vi "HGF_DSCmonitor_deregister.vi"(0 "HGF_DSCMonitor in":refnum<class "HGF_DSCMonitor.lvclass">, 1 "SV":refnum<k21>, 3 "HGF_NetworkVisitor":refnum<class "HGF_NetworkVisitor.lvclass">, 4 "HGF_TriggeredEvent":refnum<class "HGF_TriggeredEvent.lvclass">, 5 "error in (no error)":errorcluster, 9 "Rem SV/Visitor from List":bool) -> (14 "HGF_DSCMonitor out":refnum<class "HGF_DSCMonitor.lvclass">, 19 "error out":errorcluster)   [LabVIEW 2012, in "HGF_DSC.lvlib" / "HGF_DSCMonitor.lvclass"]
uses:
  HGF_DSCMonitor.lvclass
  HGF_BaseClasses/HGF_NetworkVisitor/HGF_NetworkVisitor.lvclass
  HGF_BaseClasses/HGF_TriggeredEvent/HGF_TriggeredEvent.lvclass
  HGF_DSCMonitor.lvclass/HGF_DSCMonitor.ctl
  <vilib>/lvdsc/NI_DSC.lvlib
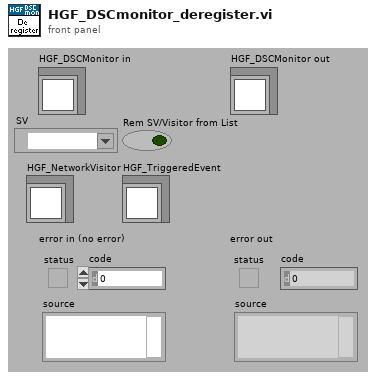
[diagram p1: front panel]
types:
  T1 = cluster{"Shared Variable":refnum<k21>, "registered Visitors":cluster{"HGF_NetworkVisitor":refnum<class "HGF_NetworkVisitor.lvclass">, "HGF_TriggeredEvent":refnum<class "HGF_TriggeredEvent.lvclass">}[]}[]
  T2 = cluster{"HGF_NetworkVisitor":refnum<class "HGF_NetworkVisitor.lvclass">, "HGF_TriggeredEvent":refnum<class "HGF_TriggeredEvent.lvclass">}
  T3 = cluster{"Shared Variable":refnum<k21>, "registered Visitors":cluster{"HGF_NetworkVisitor":refnum<class "HGF_NetworkVisitor.lvclass">, "HGF_TriggeredEvent":refnum<class "HGF_TriggeredEvent.lvclass">}[]}
  T4 = cluster{"HGF_NetworkVisitor":refnum<class "HGF_NetworkVisitor.lvclass">, "HGF_TriggeredEvent":refnum<class "HGF_TriggeredEvent.lvclass">}[]
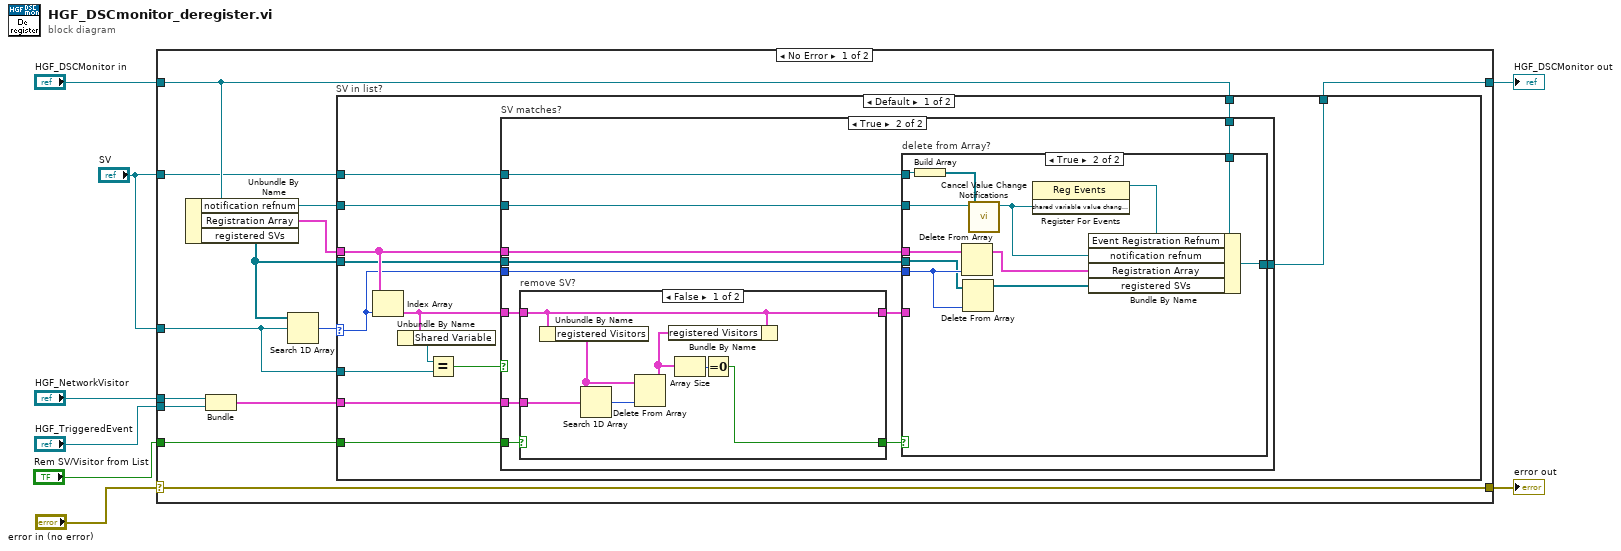
[diagram p0: block diagram]
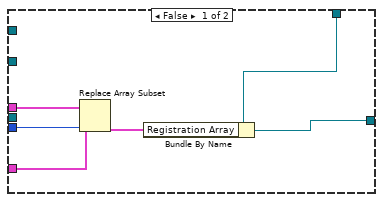
[diagram p3: hidden frame]
diagram:
  n1 = case shown="No Error" "error in (no error)" {
    selector: "error in (no error)" -> [w21 w76]
    tunnel: [w21 w76] -> w7
    tunnel: [w11 w75] -> w5
    tunnel: "HGF_DSCMonitor in" -> [w12 w75]
    tunnel: "SV" -> [w16 _]
    tunnel: "HGF_TriggeredEvent" -> [w18 _]
    tunnel: "HGF_NetworkVisitor" -> [w17 _]
    tunnel: "Rem SV/Visitor from List" -> [w14 _]
    tunnel: "SV" -> [w9 _]
    frame No Error {
      n2 = Unbundle By Name(w12) -> ("notification refnum"=w10:refnum<user-event>, "Registration Array"=w19:T1, "registered SVs"=w13:refnum<k21>[])
      n3 = Bundle("HGF_NetworkVisitor"=w17, "HGF_TriggeredEvent"=w18) -> (w15:T2)  [unwired: 1 out]
      n4 = Search 1D Array(1D array=w13, element=w16) -> (index of element=w20:i32)  [unwired: 1 out]
      n5 = case "SV in list?" shown="Default" w20 {
        selector: w20 -> [w27 _]
        tunnel: w19 -> [w28 _]
        tunnel: w16 -> [w33 _]
        tunnel: w15 -> [w30 _]
        tunnel: w14 -> [w29 _]
        tunnel: w13 -> [w26 _]
        tunnel: w12 -> [w25 w74]
        tunnel: [w24 w74] -> w11
        tunnel: w10 -> [w23 _]
        tunnel: w9 -> [w22 _]
        frame Default {
          n6 = Index Array(array=w28, index=w27) -> (element=w31:T3)
          n7 = Unbundle By Name(w31) -> ("Shared Variable"=w34:refnum<k21>)
          n8 = Equal?(x=w34, y=w33) -> (x = y?=w32:bool)
          n9 = case "SV matches?" shown="True" w32 {
            tunnel: w31 -> [_ w46]
            tunnel: w30 -> [_ w47]
            tunnel: w29 -> [_ w45]
            tunnel: w28 -> [_ w43]
            tunnel: w27 -> [_ w41]
            tunnel: w26 -> [_ w40]
            tunnel: w25 -> [w35 w39]
            tunnel: [w35 w38] -> w24
            tunnel: w23 -> [_ w37]
            tunnel: w22 -> [_ w36]
            frame False {
            }
            frame True {
              n10 = case "remove SV?" shown="False" w45 {
                selector: w45 -> [_ w73]
                tunnel: w47 -> [w72 _]
                tunnel: w46 -> [w66 _]
                tunnel: [w67 w73] -> w44
                tunnel: [w66 _] -> w42
                frame False {
                  n11 = Unbundle By Name(w66) -> ("registered Visitors"=w70:T4)
                  n12 = Search 1D Array(1D array=w70, element=w72) -> (index of element=w71:i32)  [unwired: 1 out]
                  n13 = Delete From Array(array=w70, index=w71) -> (array with subset deleted=w69:T4)  [unwired: 1 in, 1 out]
                  n14 = Bundle By Name(cluster=w66, "registered Visitors"=w69) -> ()  [unwired: 1 out]
                  n15 = Array Size(array=w69) -> (size(s)=w68:i32)
                  n16 = Equal To 0?(x=w68) -> (x = 0?=w67:bool)
                }
                frame True {
                }
              }
              n17 = case "delete from Array?" shown="True" w44 {
                tunnel: w43 -> [w53 w65]
                tunnel: w42 -> [w51 _]
                tunnel: w41 -> [w52 w64]
                tunnel: w40 -> [_ w59]
                tunnel: w39 -> [w50 w63]
                tunnel: [w48 w60] -> w38
                tunnel: w37 -> [_ w57]
                tunnel: w36 -> [_ w58]
                frame False {
                  n18 = Replace Array Subset(array=w53, new element=w51, index=w52) -> (w49:T1)
                  n19 = Bundle By Name(cluster=w50, "Registration Array"=w49) -> (w48:refnum<class "HGF_DSCMonitor.lvclass">)
                }
                frame True {
                  n20 = Build Array(w58) -> (w56:refnum<k21>[])
                  n21 = Delete From Array(array=w65, index=w64) -> (array with subset deleted=w62:T1)  [unwired: 1 in, 1 out]
                  n22 = Delete From Array(array=w59, index=w64) -> (array with subset deleted=w61:refnum<k21>[])  [unwired: 1 in, 1 out]
                  n23 = call <vilib>:"Cancel Value Change Notifications.vi"("shared variables"=w56, "notification refnum"=w57) -> ("shared variable value change notification"=w55:refnum<user-event>)  [unwired: 1 in, 8 out]
                  n24 = register-events(w55) -> (reference out=w54:refnum<event-registration>)  [unwired: 2 in, 1 out]
                  n25 = Bundle By Name(cluster=w63, "Event Registration Refnum"=w54, "notification refnum"=w55, "Registration Array"=w62, "registered SVs"=w61) -> (w60:refnum<class "HGF_DSCMonitor.lvclass">)
                }
              }
            }
          }
        }
        frame -1 {
        }
      }
    }
    frame Error {
    }
  }
  "error out" <- w7
  "HGF_DSCMonitor out" <- w5
